vi "GetFont.vi"(8 "error in (no error)":errorcluster, 11 "menu in":refnum<class "menu.lvclass">) -> (0 "error out":errorcluster, 2 "font":cluster{"name":string, "size":i16, "color":u32}, 3 "menu out":refnum<class "menu.lvclass">)   [LabVIEW 2009, in "menu.lvclass"]
uses:
  menu.lvclass
  menu.lvclass/menu.ctl
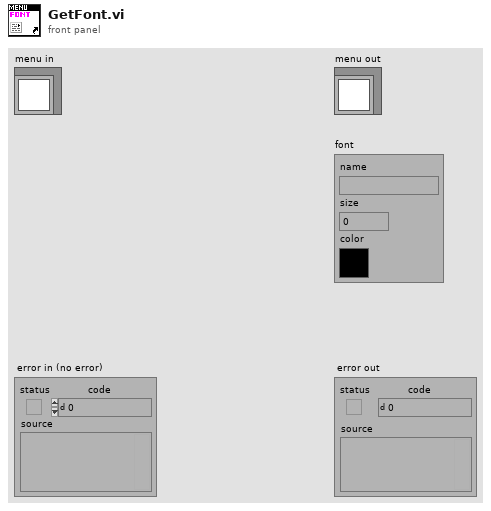
[diagram p1: front panel]
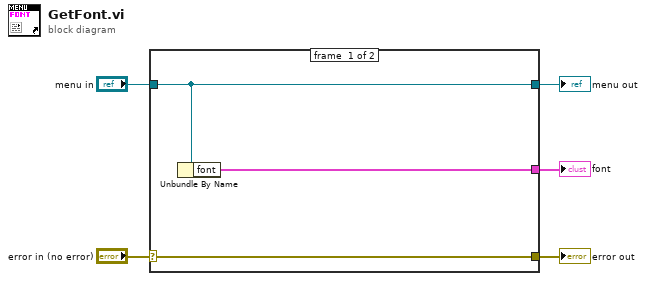
[diagram p0: block diagram]
diagram:
  n1 = case shown="No Error" "error in (no error)" {
    selector: "error in (no error)" -> [w8 w9]
    tunnel: [w8 w9] -> w2
    tunnel: [w7 w10] -> w4
    tunnel: "menu in" -> [w7 w10]
    tunnel: [w6 _] -> w1
    frame #0 {
      n2 = Unbundle By Name(w7) -> ("font"=w6:cluster{"name":string, "size":i16, "color":u32})
    }
    frame #1 {
    }
  }
  "error out" <- w2
  "menu out" <- w4
  "font" <- w1
